vi "CreateManyFiles.vi"(4 "error in":errorcluster, 6 "NumFiles":i32=100, 7 "Folder name":string) -> (0 "error out":errorcluster, 2 "Elapsed Time (ms)":u32, 3 "created path":path)   [LabVIEW 2017]
panel:
  # "Creates subdirectory of home"
  # "Creates this many empty .txt files in that directory"
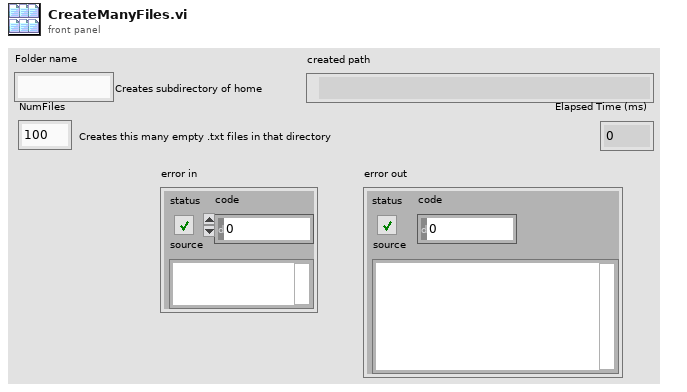
[diagram p1: front panel]
types:
  T1 = enum16{"open", "replace", "create", "open or create", "replace or create", "replace or create with confirmation"}
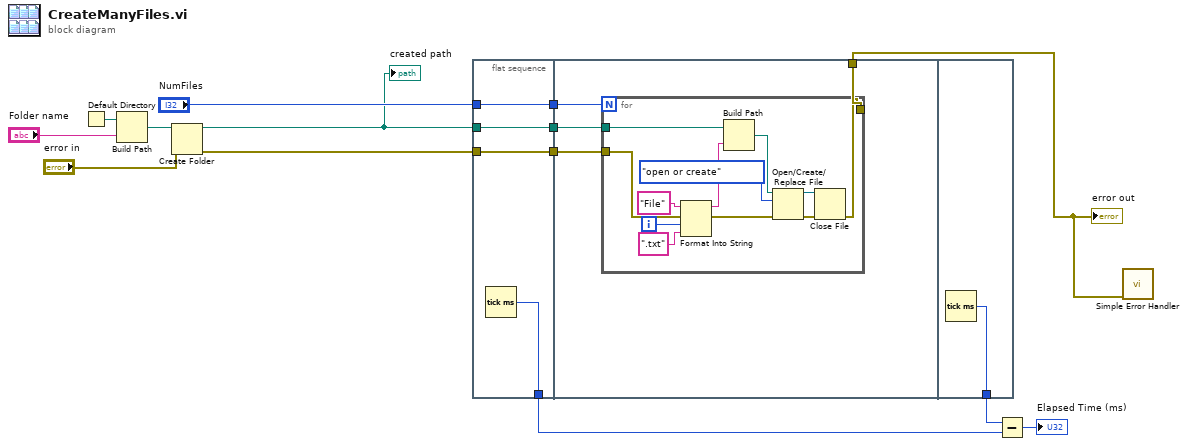
[diagram p0: block diagram]
diagram:
  n1 = Default Directory() -> (w14:path)
  n2 = Build Path(base path=w14, name or relative path="Folder name") -> (appended path=w10:path)
  n3 = Create Folder(path (use dialog)=w10, error in="error in") -> (created path=w11:path, error out=w8:errorcluster)  [unwired: 1 in, 1 out]
  "created path" <- w11
  n4 = flat-sequence {
    tunnel: w8 -> [w16]
    tunnel: w11 -> [w17]
    tunnel: "NumFiles" -> [w18]
    tunnel: [w18] -> w7
    tunnel: [w17] -> w6
    tunnel: [w16] -> w5
    tunnel: [w15] -> w3
    tunnel: w7 -> [w22]
    tunnel: w6 -> [w21]
    tunnel: w5 -> [w20]
    tunnel: [w19] -> w1
    tunnel: [w35] -> w4
    frame #0 {
      n5 = Tick Count (ms)() -> (millisecond timer value=w15:u32)
    }
    frame #1 {
      n6 = for {
        N: w22 -> [_]
        tunnel: w21 -> [w33]
        tunnel: w20 -> [w24]
        tunnel: [w23] -> w19
        i -> [w30]
        n7 = Format Into String(initial string="File", error in=w24, w30, ".txt") -> (resulting string=w32:string, error out=w28:errorcluster)  [unwired: 1 in]
        n8 = Build Path(base path=w33, name or relative path=w32) -> (appended path=w27:path)
        n9 = Open/Create/Replace File(file path (use dialog)=w27, error in=w28, operation (0:open)=T1."open or create") -> (refnum out=w26:refnum<file>, error out=w25:errorcluster)  [unwired: 3 in, 1 out]
        n10 = Close File(refnum=w26, error in=w25) -> (error out=w23:errorcluster)  [unwired: 1 out]
      }
    }
    frame #2 {
      n11 = Tick Count (ms)() -> (millisecond timer value=w35:u32)
    }
  }
  n12 = Subtract(x=w4, y=w3) -> (x-y=→"Elapsed Time (ms)":u32)
  n13 = call <vilib>:"Simple Error Handler.vi"("error in (no error)"=w1) -> ()  [unwired: 4 in, 5 out]
  "error out" <- w1
